vi "pid_control_labview.vi"() -> ()   [LabVIEW 2021]
uses:
  <vilib>/Simulation/Scripting/Companion Diagram/SimConfigNode/SimParams.ctl
  <vilib>/Simulation/Scripting/Companion Diagram/SimConfigNode/_simSolvers.ctl
  <vilib>/Simulation/Implementation/Shared/SIMSCR Execution Mode.ctl
  <vilib>/Simulation/Param Hierarchy/Typedefs/SIMPH Param Control Actions.ctl
  <vilib>/Simulation/Scripting/Editor Utilities/SIM subVI tag data.ctl
  <vilib>/Simulation/Scripting/Editor Utilities/SIM subVI execution type.ctl
  <vilib>/Simulation/Implementation/Shared/NILVSim_ParamChanged.vi
  <vilib>/Simulation/Implementation/Shared/NILVSim_FinishedLate.vi
  <vilib>/Simulation/Implementation/Shared/NILVSIM_BeginStep.vi
  <vilib>/Simulation/Utility/Implementation/SIM Halt.vi
  <vilib>/Simulation/Implementation/Shared/SIM Is Init or Final Stage.vi
  <vilib>/Simulation/ContinuousLinear/Implementation/NILVSim Transfer Function.llb/SIM Transfer Function Distributor (SISO).vi
  <vilib>/Analysis/5stat.llb/Polynomial Interpolation.vi
  <vilib>/Simulation/SignalDisplay/Implementation/NILVSim Time Waveform.llb/SIM Time Waveform (vector).vi
  <vilib>/Simulation/Implementation/Shared/SIM Fire Discrete SubVI.vi
  <vilib>/Simulation/SignalDisplay/Implementation/NILVSim Time Waveform.llb/SIM Time Waveform (scalar).vi
  <vilib>/Simulation/ContinuousLinear/Implementation/NILVSim Transfer Function.llb/SIM Transfer Function Collector (SISO).vi
  <vilib>/Simulation/Implementation/Shared/NILVSim_Manager.vi
  <vilib>/Utility/error.llb/Clear Errors.vi
  <vilib>/Simulation/Implementation/Shared/NILVSim_FinalizeModel.vi
  <vilib>/Simulation/Implementation/Shared/SIM Fire Discrete SubVI (Core).vi
  <vilib>/Simulation/Implementation/Shared/SIM Unbundle Sim Info.vi
  <vilib>/Simulation/Implementation/Shared/SIMSH Read Queue.vi
  <vilib>/Simulation/Implementation/Shared/NILVSim_Initialize.vi
  <vilib>/ptbypt/Signal Generation.llb/Uniform White Noise PtByPt.vi
  timeconstant_lowpass_filter.vi
  <vilib>/addons/control/pid/pid.llb/PID Advanced.vi
  <vilib>/addons/control/pid/pid.llb/PID Advanced (DBL).vi
  <vilib>/Simulation/Utility/Implementation/NILVSim Get Time and IsAcceptedStep.vi
  <vilib>/Simulation/Implementation/Shared/NILVSim_GetModelError.vi
  <vilib>/Simulation/Implementation/Shared/SIM Bundle Sim Info.vi
  <vilib>/Simulation/Scripting/Companion Diagram/SimConfigNode/SimDog.xnode
  <vilib>/Simulation/Implementation/XNodeFramework/SimXNode/SimX.xnode
  <vilib>/addons/control/pid/NI_PID_pid.lvlib
  <vilib>/Analysis/NI_AALPro.lvlib
  <vilib>/ptbypt/NI_PtbyPt.lvlib
  <vilib>/Simulation/ContinuousLinear/Implementation/NILVSim Transfer Function.llb/SIM Transfer Function (SISO).vi
  <vilib>/Simulation/Implementation/Shared/NI_SIM_Implementation.lvlib
panel:
  in  "Reinitialize\ncontroller":bool
  out "Waveform Chart u":waveform(dbl)(graph)={"t0"=timestamp(11.55 s since 1904-01-01), "dt"=1.0, "Y"=[1.162858812206253]}
  in  "Sim/Real?":bool caption="Connect to simulated or real process:"
  out "Waveform Chart y":waveform(dbl)[](graph)=[{"t0"=timestamp(11.55 s since 1904-01-01), "dt"=1.0, "Y"=[2.0]}, {"t0"=timestamp(11.55 s since 1904-01-01), "dt"=1.0, "Y"=[2.067853538426915]}, {"t0"=timestamp(11.55 s since 1904-01-01), "dt"=1.0, "Y"=[2.0166383987927947]}]
  in  "Physical_min_max [kRPM]":dbl[](array[numeric])=[-5.0, 5.0] format="%0.2f"
  in  "Meas_min_max [V]":dbl[](array[numeric])=[-10.0, 10.0] format="%0.2f"
  in  "Filter time-constant\nTf [s]":dbl=0.2
  in  "Time step Ts [s]":dbl=0.05
  in  "Setpoint y_SP\n[kRPM]":dbl(slide)=2.0 scale=-5.0..5.0 scale format="%.2f"
  in  "Auto/Man?":bool=TRUE
  in  "u_man [V]":dbl
  in  "Controller output (u)\nrange [V]":cluster{"Output high":dbl, "Output low":dbl}={"Output high"=10.0, "Output low"=-10.0}
  in  "Setpoint (y_SP)\nrange [kRPM]":cluster{"Setpoint high":dbl, "Setpoint low":dbl}={"Setpoint high"=5.0, "Setpoint low"=-5.0}
  in  "PID gains":T1={"Proportional gain Kc"=3.0, "Integral time Ti [sec]"=2.0, "Derivative time Td [sec]"=0.0}
  in  "stop":bool
  # "PID Control System"
  # "By Finnn Haugen"
  # "finn@techteach.no"
  # "1. March 2008"
  # "Auto"
  # "Connect to simulated or real process:"
  # "Sim"
  # "Real (if there was one)"
  # "Man"
  # "(Process is an assumed motor incl speed sensor\nwith gain 0.5 and time-constant 2 sec. Measurement\nnoise is included in the simulated process.)"
  # "y_SP [kRPM]"
  # "y [V]"
  # "u [V]"
  # "Process\nincl.\nsensor"
  # "PID\nController"
  # "Simulated/real"
  # "Lowpass\nFilter"
  # "Scaling"
  # "y_filt [kRPM]"
  # "y [kRPM]"
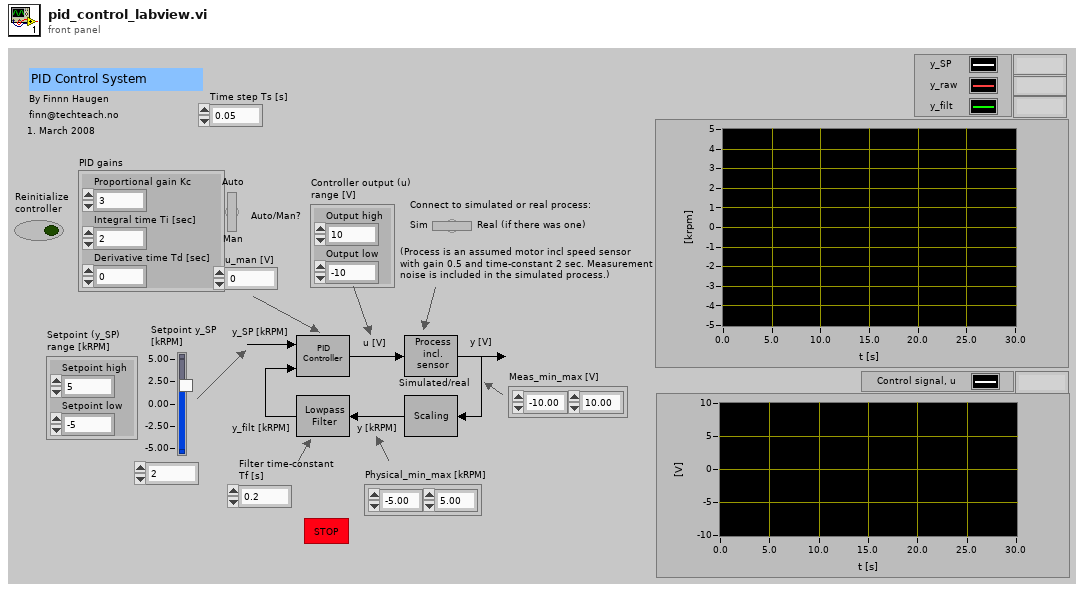
[diagram p1: front panel]
types:
  T1 = cluster{"Proportional gain Kc":dbl, "Integral time Ti [sec]":dbl, "Derivative time Td [sec]":dbl}
  T2 = enum16{"Runge-Kutta 1 (Euler)", "Runge-Kutta 2", "Runge-Kutta 3", "Runge-Kutta 4", "Runge-Kutta 23 (variable)", "Runge-Kutta 45 (variable)", "BDF (variable)", "Adams-Moulton (variable)", "Rosenbrock (variable)", "Discrete States Only"}
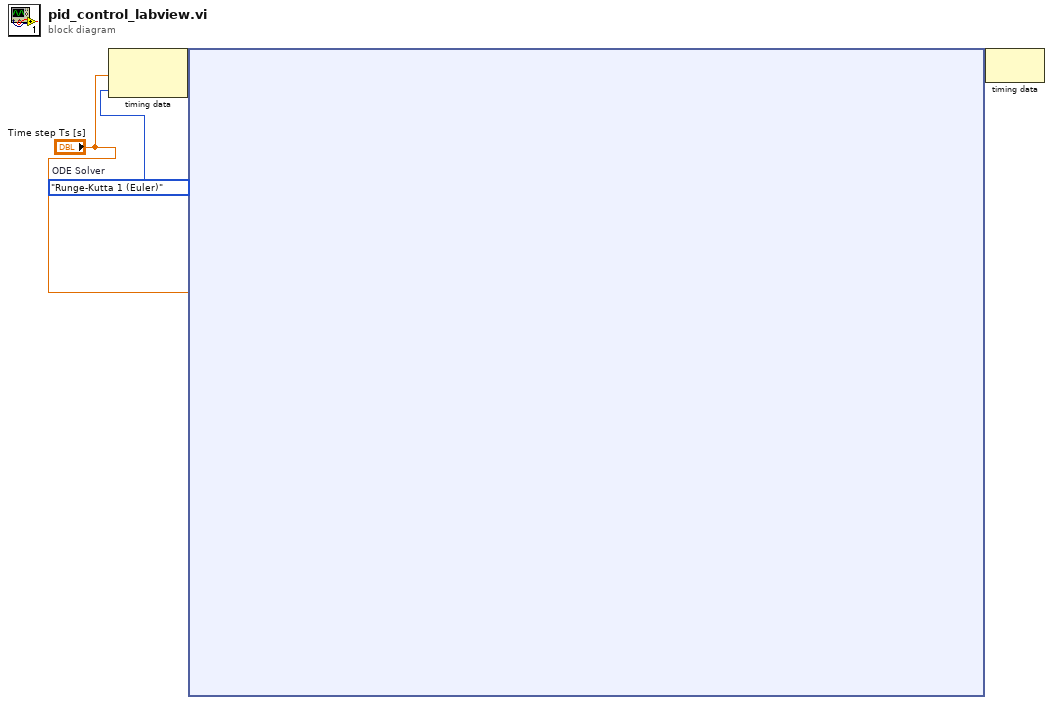
[diagram p0: block diagram]
diagram:
  w2 = T2."Runge-Kutta 1 (Euler)"  # ODE Solver
  n1 = node-c288("Time step Ts [s]", w2) -> (w4:variant)
  n2 = node-c254 ("Control & Simulation Loop")(w4, "Time step Ts [s]") -> (w3:variant)
  n3 = node-c288(w3) -> ()  [unwired: 1 out]
